vi "Network Sink Test Panel.vi"() -> ()   [LabVIEW 2017]
uses:
  <vilib>/gpm_packages/@cs/event-logger/Source/Composed Log/LoggerReference/LoggerReference.lvclass/LoggerReference.ctl
  <vilib>/gpm_packages/@cs/event-logger/Source/Composed Log/Types/Log Level.ctl
  13a051d5-a32e-4c76-9e98-7aaf70981655.vi
  b558ab63-4aa2-4cbd-b208-fa7bab295c73.vi
  8cfab7ac-fb16-44d0-a6dd-ea15f75b8495.vi
  <vilib>/gpm_packages/@cs/event-logger/Source/Composed Log/LoggerReference/Return Aggregate Queues.vi
  <vilib>/gpm_packages/@cs/event-logger/Source/Composed Log/LoggerReference/Add Aggregate Log.vi
  13a051d5-a32e-4c76-9e98-7aaf70981655.vi/57ccd4d0-4ce1-447b-bbd8-0792d13e6155.vi
  b558ab63-4aa2-4cbd-b208-fa7bab295c73.vi/e2a7d12d-3fc5-4ec8-b3d7-7ff867e414fe.vi
  <vilib>/gpm_packages/@cs/event-logger/Source/Composed Log/LoggerReference/Log.vi
  <vilib>/gpm_packages/@cs/event-logger/Source/Composed Log/LoggerReference/Get Valid Event Time.vi
  <vilib>/gpm_packages/@cs/event-logger/Source/Composed Log/LoggerReference/Send Add Sink.vi
  <vilib>/gpm_packages/@cs/event-logger/Source/Composed Log/LoggerReference/Remove Stale Logs.vi
  <vilib>/gpm_packages/@cs/event-logger/Source/String Control Sink/String Control Sink.lvclass
  C:/Program Files/National Instruments/LabVIEW 2017/vi.lib/gpm_packages/@cs/event-logger/Source/Composed Log/Log Sink/Log Sink.lvclass
  <vilib>/gpm_packages/@cs/Network-sink/Source/Network Sink/Network Sink/Network Sink.lvclass
  <vilib>/gpm_packages/@cs/event-logger/Source/Composed Log/Application Logger/Launch Worker Loop.vi
  <vilib>/gpm_packages/@cs/event-logger/Source/Composed Log/LoggerReference/Initialize Logger Instance.vi
  <vilib>/gpm_packages/@cs/event-logger/Source/Composed Log/LoggerReference/LoggerReference.lvclass
  <vilib>/gpm_packages/@cs/event-logger/Source/Composed Log/IErrorFormat/IErrorFormat.lvclass
  <vilib>/gpm_packages/@cs/event-logger/Source/Composed Log/Log Sink/Log Sink.lvclass
  <vilib>/gpm_packages/@cs/event-logger/Source/Composed Log/Composed Log.lvlib
  <vilib>/gpm_packages/@cs/Network-sink/Source/Network Sink/Network Sink Endpoint/Network Sink Endpoint.lvclass
panel:
  in  "Remote Event Log":string
  in  "Local Event Log":string
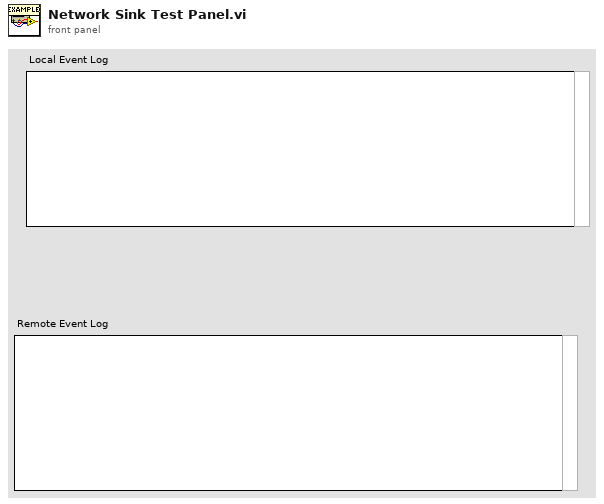
[diagram p1: front panel]
types:
  T1 = typedef "Composed Log.lvlib/Log Level.ctl" = enum16{"Debug", "Info", "Warning", "Error", "Critical"}
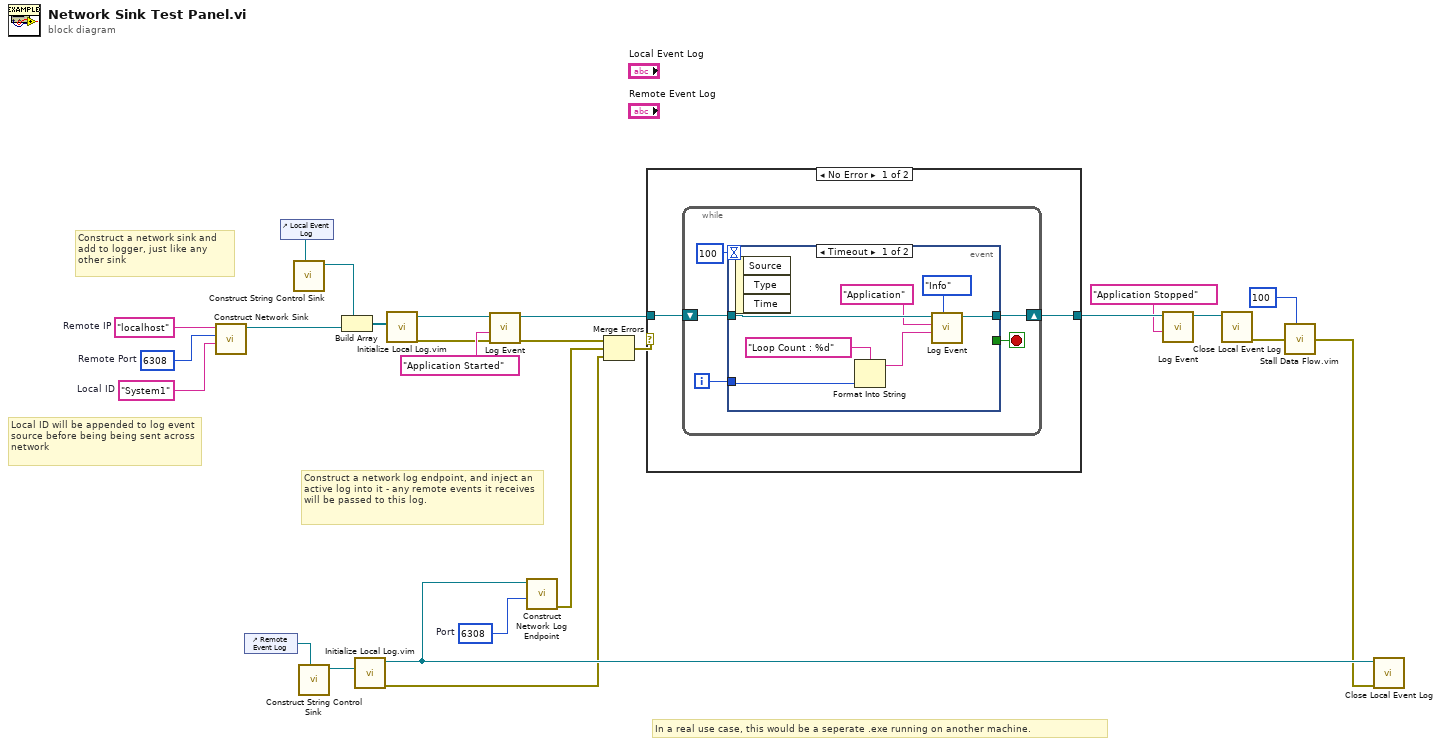
[diagram p0: block diagram]
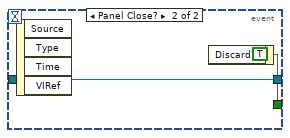
[diagram p2: hidden frame]
diagram:
  w17 = u16 6308  # Port
  w20 = u16 6308  # Remote Port
  w21 = "System1"  # Local ID
  w22 = "localhost"  # Remote IP
  # "In a real use case, this would be a seperate .exe running on another machine."
  # "Construct a network log endpoint, and inject an active log into it - any remote events it receives will be passed to this log."
  # "Construct a network sink and add to logger, just like any other sink"
  # "Local ID will be appended to log event source before being being sent across network"
  n1 = call <vilib>:"Construct Network Sink.vi"("Local ID"=w21, "Remote Port"=w20, "Remote IP"=w22) -> ("Network Sink out"=w13:refnum<class "Network Sink.lvclass">)  [unwired: 8 in]
  n2 = control-ref of="Remote Event Log"() -> (w19:refnum<vi>)
  n3 = control-ref of="Local Event Log"() -> (w24:refnum<vi>)
  n4 = call <vilib>:"Construct String Control Sink.vi"("Str Refnum"=w24) -> ("String Control Sink out"=w25:refnum<class "String Control Sink.lvclass">)  [unwired: 10 in]
  n5 = call <vilib>:"Construct String Control Sink.vi"("Str Refnum"=w19) -> ("String Control Sink out"=w18:refnum<class "String Control Sink.lvclass">)  [unwired: 10 in]
  n6 = Build Array(w25, w13) -> (w23:refnum<class "Log Sink.lvclass">[])
  n7 = call "Initialize Local Log.vim"("Startup Sink(s)"=w18) -> ("error out"=w3:errorcluster, "Log Instance Reference"=w7:refnum<class "LoggerReference.lvclass">)  [unwired: 8 in, 1 out]
  n8 = call "Initialize Local Log.vim"("Startup Sink(s)"=w23) -> ("error out"=w8:errorcluster, "Log Instance Reference"=w11:refnum<class "LoggerReference.lvclass">)  [unwired: 8 in, 1 out]
  n9 = call <vilib>:"Log Event.vi"("error in (no error)"=w8, "Data To Log"="Application Started", "Log Instance"=w11) -> ("error out"=w9:errorcluster, "Log Instance Out"=w10:refnum<class "LoggerReference.lvclass">)  [unwired: 7 in]
  n10 = call <vilib>:"Construct Network Log Endpoint.vi"("Port"=w17, "Logger to Write To"=w7) -> ("error out"=w4:errorcluster)  [unwired: 8 in, 1 out]
  n11 = Merge Errors(w9, w4, w3) -> (w5:errorcluster)
  n12 = case shown="No Error" w5 {
    tunnel: w10 -> [w27 w42]
    tunnel: [w26 w42] -> w16
    frame No Error {
      n13 = while {
        shift-right: [w30] -> w26
        shift-left: w27 -> [w31]
        i -> [w28]
        stop <- w32 stop-if-true
        n14 = event shown="[0] Timeout" {
          selector: _ -> [_ _]
          dyn-events: _ -> [_ _]
          timeout: 100 -> [_ _]
          tunnel: [_ w41] -> w32
          tunnel: w31 -> [w39 w40]
          tunnel: [w37 w40] -> w30
          tunnel: w28 -> [w35 _]
          event Timeout {
            n15 = event-data() -> ()  [unwired: 1 in, 3 out]
            n16 = Format Into String(format string="Loop Count : %d" ("Data To Log"), w35) -> (resulting string=w33:string)  [unwired: 2 in, 1 out]
            n17 = call <vilib>:"Log Event.vi"("Event Level"=Log_Level."Info", "Data To Log"=w33, "SourceID"="Application", "Log Instance"=w39) -> ("Log Instance Out"=w37:refnum<class "LoggerReference.lvclass">)  [unwired: 6 in, 1 out]
          }
          event Panel Close? {
            w41 = TRUE ("Discard?")
            n18 = event-data() -> ()  [unwired: 1 in, 4 out]
            n19 = event-data("Discard?"=w41) -> ()  [unwired: 1 in, 1 out]
          }
        }
      }
    }
    frame Error {
    }
  }
  n20 = call <vilib>:"Log Event.vi"("Data To Log"="Application Stopped", "Log Instance"=w16) -> ("Log Instance Out"=w15:refnum<class "LoggerReference.lvclass">)  [unwired: 8 in, 1 out]
  n21 = call <vilib>:"Close Local Event Log.vi"("Log Instance"=w15) -> ("error out"=w6:errorcluster)  [unwired: 10 in]
  n22 = call "Stall Data Flow.vim"("value in"=w6, "milliseconds to wait"=u32 100) -> ("value out"=w2:errorcluster)  [unwired: 1 out]
  n23 = call <vilib>:"Close Local Event Log.vi"("error in (no error)"=w2, "Log Instance"=w7) -> ()  [unwired: 9 in, 1 out]
